vi "RT Driver VI.vi"(6 "Device Clock":string, 9 "Device Inputs FIFO":refnum<k33>, 10 "Device Outputs FIFO":refnum<k33>, 11 "Device Reference":T1 format="%.0x") -> ()   [LabVIEW 2019, in "TimingDRV Engine.lvlib"]
uses:
  TimingDRV Engine.lvlib
  <vilib>/NI VeriStand/Custom Device API/Custom Device Item Ref.ctl
  Parent Classes/Process/TypeDefs/Async Paramters.ctl
  <vilib>/NI VeriStand/Custom Device API/Custom Device Engine Event Ref.ctl
  <vilib>/NI VeriStand/Custom Device API/Message (Byte Array).ctl
  <vilib>/NI VeriStand/Custom Device API/Message Response (Byte Array).ctl
  <vilib>/NI VeriStand/Custom Device API/Message (String).ctl
  <vilib>/NI VeriStand/Custom Device API/Message Response (String).ctl
  Processes/Random Process/Random Process.lvclass
  Processes/Sine Process/Sine Process.lvclass
  Parent Classes/Process/Process.lvclass
  Assembler/TypeDefs/Assembler Configuration.ctl
  Assembler/TypeDefs/Process Configuration.ctl
  Assembler/Assembler.lvclass
  <vilib>/NI VeriStand/Custom Device API/Get Item Property (String).vi
  <vilib>/NI Veristand/Custom Device Tools/Custom Device Utility Library/Custom Device Utility Library.lvlib
  <vilib>/NI VeriStand/Custom Device API/Custom Device API.lvlib
panel:
  in  "Initialization Status Notifier":refnum<notifier>
  in  "Status Notifier":refnum<notifier>
  # "Custom Device Template\nv1.0"
  # "Use this template as a starting point for creating a custom device code module. The input controls shown here are specially named controls that the system will use to provide the device loop with data. The controls are not required for the device loop to run. For instance, if the device doesn't produce any output data, then you don't need the Device Outputs FIFO control. If you do use these controls, however, they need to have these exact names to be functional."
  # "The optional status notifier element is used to notify the RT engine of the last state of the custom device, and to indicate the device has completed execution. If this control is not used, a default No Error value is returned to the system when the device finishes execution.\n\nNote: This error state is not checked until the system shuts down. Use an output status channel to send more immediate status values to the system."
  # "This optional input can be used to send the VeriStand Engine the final status of the custom device initalization process. If this control exists on the custom device front panel, the VeriStand Engine will wait for a status update before starting up. If the custom device reports an error, that will abort the execution of the current configuration in the VeriStand Engine.\n\nThis control can be deleted if the custom device does not need to send the initialization status update."
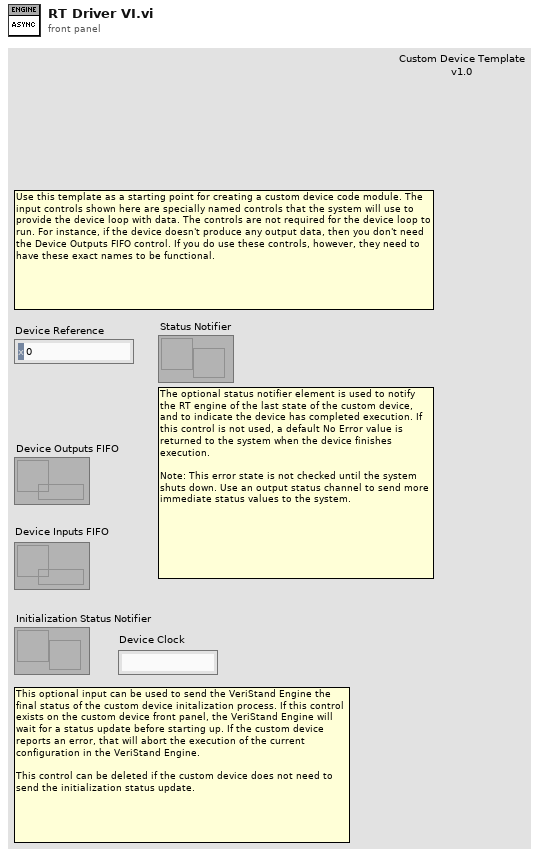
[diagram p1: front panel]
types:
  T1 = typedef "Custom Device API.lvlib/Custom Device Item Ref.ctl" = u64
  T2 = typedef "TimingDRV Engine.lvlib/Process.lvclass/Async Paramters.ctl" = cluster{"Device Reference":T1, "Device Clock":string, "Device Inputs FIFO":refnum<k33>, "Device Outputs FIFO":refnum<k33>, "CD Engine Event Ref":T3}
  T3 = typedef "Custom Device API.lvlib/Custom Device Engine Event Ref.ctl" = refnum<event-registration>
  T4 = typedef "TimingDRV Engine.lvlib/Assembler.lvclass/Assembler Configuration.ctl" = cluster{"Process Settings":T5, "Processes":refnum<class "Process.lvclass">[], "CD Engine Event Ref":T3}
  T5 = typedef "TimingDRV Engine.lvlib/Assembler.lvclass/Process Configuration.ctl" = cluster{"Process Timeout":dbl}
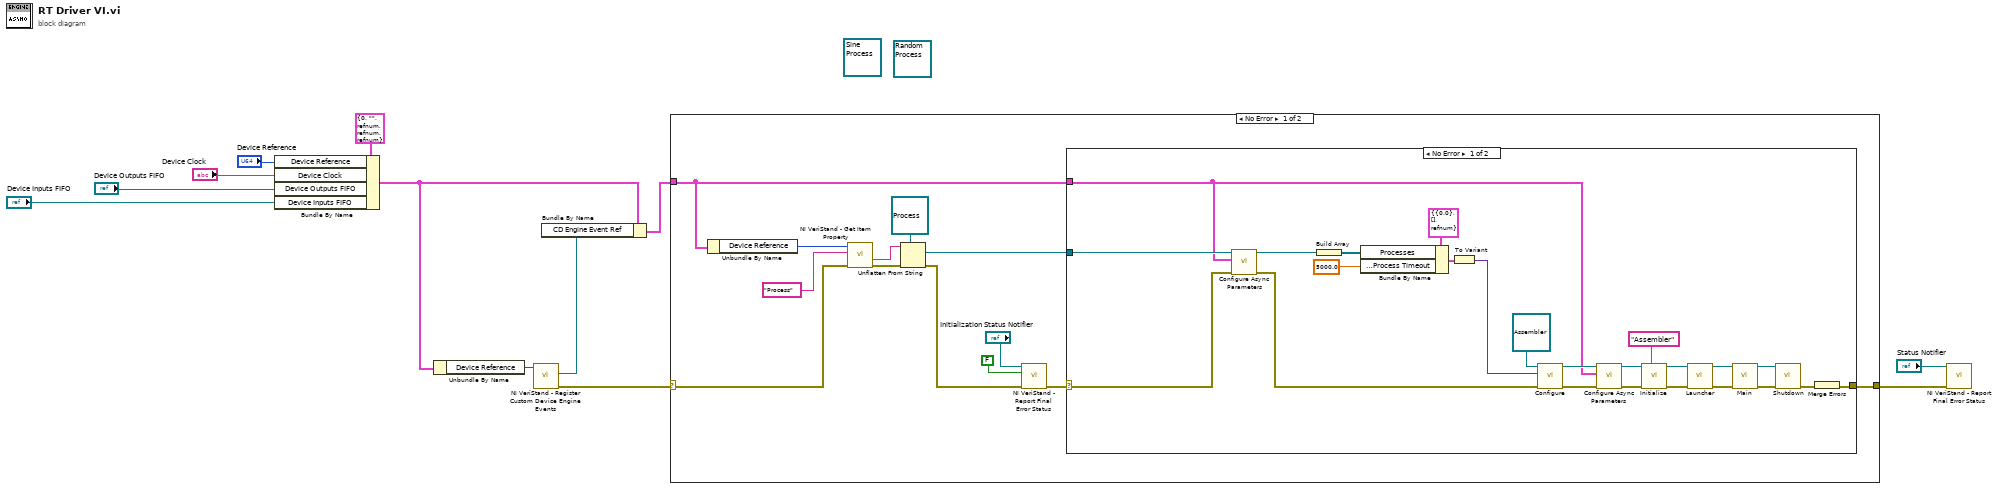
[diagram p0: block diagram]
diagram:
  (unwired) refnum<class "Sine Process.lvclass"> refnum ("TimingDRV Engine.lvlib:Sine Process.lvclass")
  (unwired) refnum<class "Random Process.lvclass"> refnum ("TimingDRV Engine.lvlib:Random Process.lvclass")
  n1 = Bundle By Name(cluster=T2 {"Device Reference"=0, "Device Clock"="", "Device Inputs FIFO"=refnum, "Device Outputs FIFO"=refnum, "CD Engine Event Ref"=refnum} ("Async Parameters"), "Device Reference"="Device Reference", "Device Clock"="Device Clock", "Device Outputs FIFO"="Device Outputs FIFO", "Device Inputs FIFO"="Device Inputs FIFO") -> (w4:T2)
  n2 = Unbundle By Name(w4) -> ("Device Reference"=w5:T1)
  n3 = call <vilib>:"NI VeriStand - Register Custom Device Engine Events.vi"("Device Ref in"=w5) -> ("error out"=w10:errorcluster, "Custom Device Engine Event Ref"=w3:T3)  [unwired: 8 in, 1 out]
  n4 = Bundle By Name(cluster=w4, "CD Engine Event Ref"=w3) -> (w2:T2)
  n5 = case shown="No Error" w10 {
    selector: w10 -> [w24 w51]
    tunnel: [w25 w51] -> w11
    tunnel: w2 -> [w15 _]
    frame No Error {
      n6 = Unbundle By Name(w15) -> ("Device Reference"=w14:T1)
      n7 = call-poly <vilib>:"NI VeriStand - Get Item Property.vi"("error in (no error)"=w24, "Property Name"="Process", "Item Ref in"=w14) -> ("error out"=w19:errorcluster, "Value"=w18:string)  [unwired: 5 in, 2 out]
      n8 = Unflatten From String(type=refnum<class "Process.lvclass"> refnum ("TimingDRV Engine.lvlib:Process.lvclass"), binary string=w18, error in (no error)=w19) -> (value=w16:refnum<class "Process.lvclass">, error out=w13:errorcluster)  [unwired: 2 in, 1 out]
      n9 = call <vilib>:"NI VeriStand - Report Final Error Status.vi"("error in (no error)"=w13, "Filter FIFO & Shutdown Errors (T)"=FALSE ("Filter FIFO Errors (T)"), "Status Notifier"="Initialization Status Notifier") -> ("error out"=w20:errorcluster)  [unwired: 8 out]
      n10 = case shown="No Error" w20 {
        selector: w20 -> [w34 w50]
        tunnel: [w37 w50] -> w25
        tunnel: w16 -> [w35 _]
        tunnel: w15 -> [w28 _]
        frame No Error {
          n11 = call-dynamic "Configure Async Parameters.vi"("error in (no error)"=w34, "Async Parameters"=w28, "Process in"=w35) -> ("error out"=w27:errorcluster, "Process out"=w33:refnum<class "Process.lvclass">)  [unwired: 7 in]
          n12 = Build Array(w33) -> (w36:refnum<class "Process.lvclass">[])
          n13 = Bundle By Name(cluster=T4 {"Process Settings"={"Process Timeout"=0.0}, "Processes"=[], "CD Engine Event Ref"=refnum} ("Assembler Configuration"), "Processes"=w36, "Process Settings.Process Timeout"=5000.0) -> (w46:T4)
          n14 = To Variant(anything=w46) -> (Variant=w45:variant)
          n15 = call-dynamic "Configure.vi"("error in (no error)"=w27, "Parameters"=w45, "Assembler in"=refnum<class "Assembler.lvclass"> refnum) -> ("error out"=w32:errorcluster, "Assembler out"=w29:refnum<class "Assembler.lvclass">)  [unwired: 7 in]
          n16 = call-dynamic "Configure Async Parameters.vi"("error in (no error)"=w32, "Async Parameters"=w28, "Process in"=w29) -> ("error out"=w31:errorcluster, "Process out"=w30:refnum<class "Assembler.lvclass">)  [unwired: 7 in]
          n17 = call-dynamic "Initialize.vi"("Process ID"="Assembler", "error in (no error)"=w31, "Assembler in"=w30) -> ("error out"=w43:errorcluster, "Assembler out"=w42:refnum<class "Assembler.lvclass">)  [unwired: 7 in]
          n18 = call-dynamic "Launcher.vi"("error in (no error)"=w43, "Assembler in"=w42) -> ("error out"=w41:errorcluster, "Assembler out"=w40:refnum<class "Assembler.lvclass">)  [unwired: 8 in]
          n19 = call-dynamic "Main.vi"("error in (no error)"=w41, "Process in"=w40) -> ("error out"=w39:errorcluster, "Process out"=w38:refnum<class "Assembler.lvclass">)  [unwired: 8 in]
          n20 = call-dynamic "Shutdown.vi"("error in (no error)"=w39, "Assembler in"=w38) -> ("error out"=w26:errorcluster)  [unwired: 9 in]
          n21 = Merge Errors(w26) -> (w37:errorcluster)
        }
        frame Error {
        }
      }
    }
    frame Error {
    }
  }
  n22 = call <vilib>:"NI VeriStand - Report Final Error Status.vi"("error in (no error)"=w11, "Status Notifier"="Status Notifier") -> ()  [unwired: 1 in, 9 out]
